vi "RFmx Analysis Only Sanity Check.vi"() -> ()   [LabVIEW 2017]
uses:
  <vilib>/Utility/error.llb/DialogType.ctl
  <vilib>/RFmx/SpecAn/mx/RFmxSpecAn.llb/RFmxSpecAn Select Measurement (Multiple).vi
  <vilib>/RFmx/SpecAn/mx/RFmxSpecAn.llb/RFmxSpecAn Analyze (IQ).vi
  <vilib>/RFmx/SpecAn/mx/RFmxSpecAn.llb/RFmxSpecAn CHP Fetch Measurement.vi
  <vilib>/RFmx/SpecAn/mx/RFmxSpecAn.llb/RFmxSpecAn TXP Fetch Power Trace.vi
  <vilib>/RFmx/SpecAn/mx/RFmxSpecAn.llb/RFmxSpecAn CHP Fetch Spectrum.vi
  <resource>/objmgr/RFmxInstr.rc
panel:
  out "Numeric Control":i32
  out "Waveform Graph":cluster{"x0":dbl, "dx":dbl, "y":sgl[]}(graph)
  in  "Enum":enum16{"Correct Behavior", "Incorrect Behavior"}(ring)
  out "Absolute Power (dBm)":dbl format="%.2f"
  out "Recommended Min Sample Rate (Hz)":dbl format="%#_6p"
  out "Recommended Acquisition Time (s)":dbl format="%#_6p"
  out "Waveform Graph 2":cluster{"x0":dbl, "dx":dbl, "y":sgl[]}(graph)
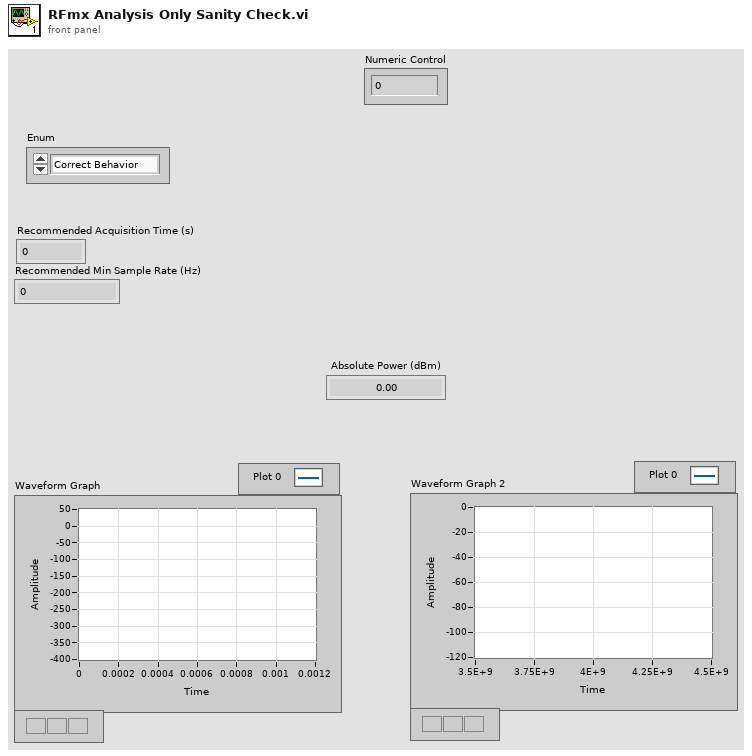
[diagram p1: front panel]
types:
  T1 = typedef "DialogType.ctl" = u16
  T2 = enum16{"open", "open or create", "create or replace", "create", "open (read-only)"}
  T3 = enum16{"ACP", "CCDF", "CHP", "FCnt", "Harmonics", "OBW", "SEM", "Spectrum", "Spur", "TXP", "AMPM", "DPD", "IQ", "IM", "NF", "PhaseNoise"}[]
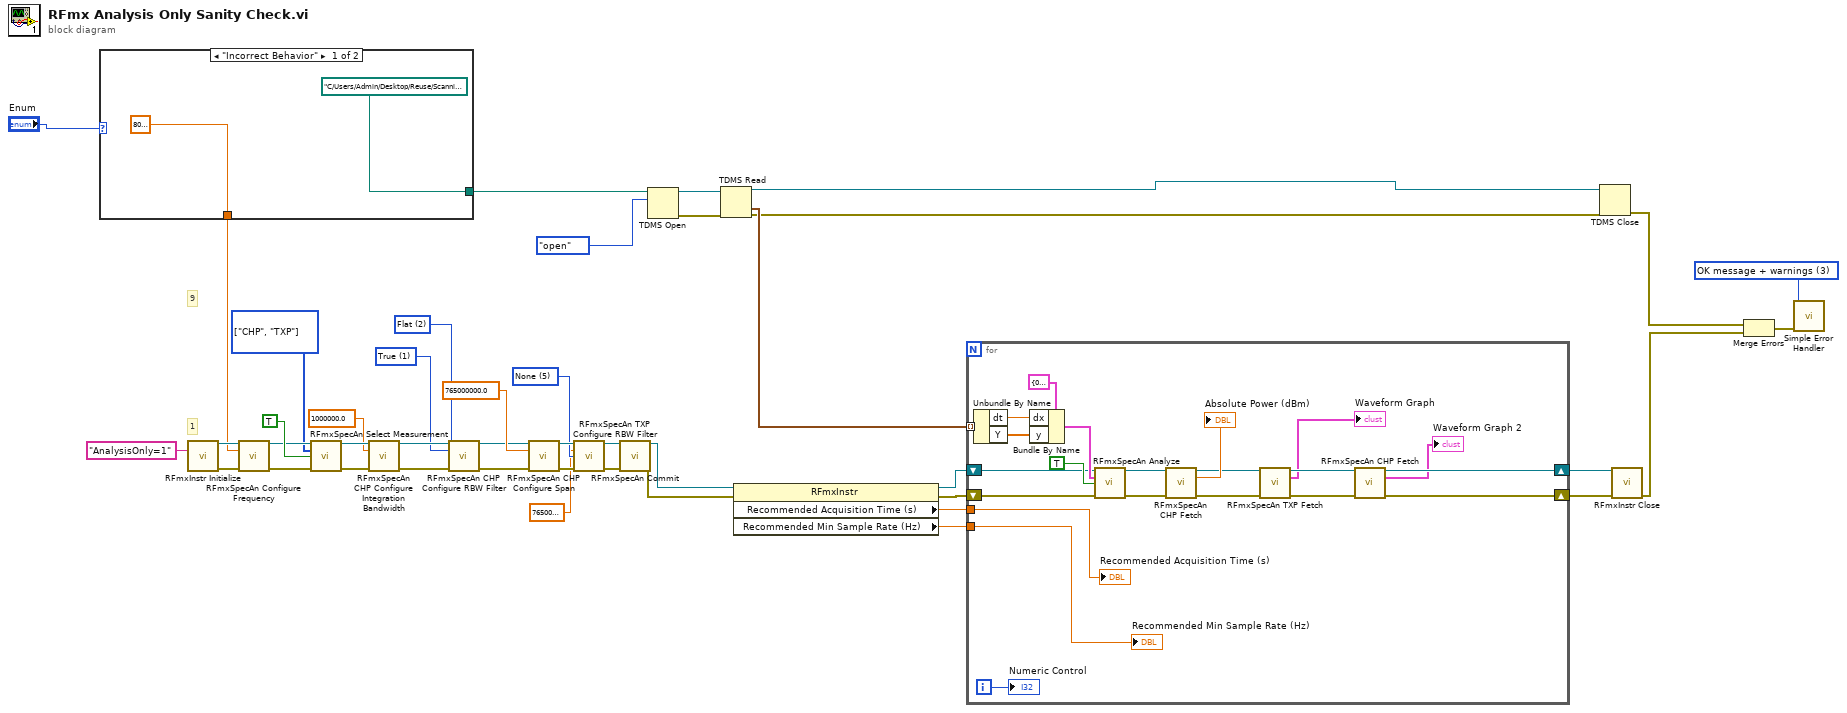
[diagram p0: block diagram]
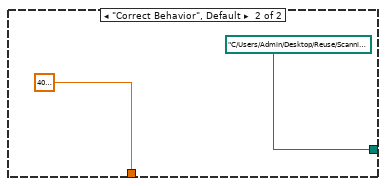
[diagram p2: hidden frame]
diagram:
  w1 = 2 items=["FFT Based", "Gaussian", "Flat"] ("RBW Filter Type")
  w2 = 1 items=["False", "True"] ("RBW Auto")
  w7 = 5 items=["None"=5, "Gaussian"=1, "Flat"=2, "RRC"=6] ("RBW Filter Type")
  w14 = T1 3 items=["no dialog", "OK message", "continue or stop message", "OK message + warnings", "continue/stop + warnings"] ("type of dialog (OK msg:1)")
  w25 = T3 [enum."CHP", enum."TXP"] items=["ACP", "CCDF", "CHP", "FCnt", "Harmonics", "OBW", "SEM", "Spectrum", "Spur", "TXP", "AMPM", "DPD", "IQ", "IM", "NF", "PhaseNoise"] ("Measurements")
  # "9"
  # "1"
  n1 = case shown="\"Incorrect Behavior\"" "Enum" {
    tunnel: [8000000000.0 ("Center Frequency (Hz)") 4000000000.0 ("Center Frequency (Hz)")] -> w26
    tunnel: [path "C:/Users/Admin/Desktop/Reuse/Scanning Speed PXIe 5668/Data8G.tdms.txt.tdms" ("file path") path "C:/Users/Admin/Desktop/Reuse/Scanning Speed PXIe 5668/Data4G.tdms.txt.tdms" ("file path")] -> w11
    frame "Incorrect Behavior" {
    }
    frame "Correct Behavior", Default {
    }
  }
  n2 = call <vilib>:"RFmxInstr Initialize.vi"("Option String"="AnalysisOnly=1") -> ("Instrument Handle Out"=w43:refnum<k21>, "error out"=w42:errorcluster)  [unwired: 12 in, 1 out]
  n3 = call <vilib>:"RFmxSpecAn Configure Frequency.vi"("Instrument Handle In"=w43, "Center Frequency (Hz)"=w26, "error in (no error)"=w42) -> ("Instrument Handle Out"=w40:refnum<k21>, "error out"=w39:errorcluster)  [unwired: 11 in]
  n4 = call-poly <vilib>:"RFmxSpecAn Select Measurement.vi"("Instrument Handle In"=w40, "Measurements"=w25, "Enable All Traces"=TRUE, "error in (no error)"=w39) -> ("Instrument Handle Out"=w38:refnum<k21>, "error out"=w37:errorcluster)  [unwired: 10 in]
  n5 = call <vilib>:"RFmxSpecAn CHP Configure Integration Bandwidth.vi"("Instrument Handle In"=w38, "Integration Bandwidth (Hz)"=1000000.0, "error in (no error)"=w37) -> ("Instrument Handle Out"=w4:refnum<k21>, "error out"=w35:errorcluster)  [unwired: 11 in]
  n6 = call <vilib>:"RFmxSpecAn CHP Configure RBW Filter.vi"("Instrument Handle In"=w4, "RBW Auto"=w2, "RBW Filter Type"=w1, "error in (no error)"=w35) -> ("Instrument Handle Out"=w3:refnum<k21>, "error out"=w5:errorcluster)  [unwired: 10 in]
  n7 = call <vilib>:"RFmxSpecAn CHP Configure Span.vi"("Instrument Handle In"=w3, "Span (Hz)"=765000000.0, "error in (no error)"=w5) -> ("Instrument Handle Out"=w9:refnum<k21>, "error out"=w30:errorcluster)  [unwired: 11 in]
  n8 = call <vilib>:"RFmxSpecAn TXP Configure RBW Filter.vi"("Instrument Handle In"=w9, "RBW (Hz)"=765000000.0, "RBW Filter Type"=w7, "error in (no error)"=w30) -> ("Instrument Handle Out"=w8:refnum<k21>, "error out"=w10:errorcluster)  [unwired: 10 in]
  n9 = call <vilib>:"RFmxSpecAn Commit.vi"("Instrument Handle In"=w8, "error in (no error)"=w10) -> ("Instrument Handle Out"=w27:refnum<k21>, "error out"=w28:errorcluster)  [unwired: 12 in]
  n10 = TDMS Open(10:T2."open" ("operation (0:open)"), 11:w11) -> (0:w21:errorcluster, 3:w20:refnum<k34>)  [unwired: 5 in]
  n11 = TDMS Read(0:w20, 11:w21) -> (4:w12:refnum<k34>, 10:w19:waveform(dbl)[], 15:w18:errorcluster)  [unwired: 6 in, 3 out]
  n12 = property class="RFmxInstr"(reference=w27, error in=w28) -> (reference out=w31:refnum<k21>, error out=w29:errorcluster, "Recommended Acquisition Time (s)"=w24:dbl, "Recommended Min Sample Rate (Hz)"=w23:dbl)
  n13 = for {
    tunnel: w24 -> [w59]
    tunnel: w23 -> [w58]
    tunnel: w19 -> [w57] mode=indexing
    shift-right: [w65] -> w33
    shift-left: w31 -> [w61]
    shift-right: [w63] -> w32
    shift-left: w29 -> [w60]
    i -> [w49]
    n14 = Unbundle By Name(w57) -> ("dt"=w56:dbl, "Y"=w55:dbl[])
    n15 = Bundle By Name(cluster=cluster{"x0":dbl, "dx":dbl, "y":csg[]} {"x0"=0.0, "dx"=0.0, "y"=[]} ("IQ"), "dx"=w56, "y"=w55) -> (w67:cluster{"x0":dbl, "dx":dbl, "y":csg[]})
    n16 = call-poly <vilib>:"RFmxSpecAn Analyze.vi"("Instrument Handle In"=w61, "IQ"=w67, "Reset?"=TRUE, "error in (no error)"=w60) -> ("Instrument Handle Out"=w70:refnum<k21>, "error out"=w69:errorcluster)  [unwired: 8 in, 2 out]
    n17 = call-poly <vilib>:"RFmxSpecAn CHP Fetch.vi"("Instrument Handle In"=w70, "error in (no error)"=w69) -> ("Instrument Handle Out"=w52:refnum<k21>, "Absolute Power (dBm)"=→"Absolute Power (dBm)":dbl, "error out"=w64:errorcluster)  [unwired: 8 in, 3 out]
    n18 = call-poly <vilib>:"RFmxSpecAn TXP Fetch.vi"("Instrument Handle In"=w52, "error in (no error)"=w64) -> ("Instrument Handle Out"=w51:refnum<k21>, "Power (dBm)"=→"Waveform Graph":cluster{"x0":dbl, "dx":dbl, "y":sgl[]}, "error out"=w53:errorcluster)  [unwired: 11 in]
    n19 = call-poly <vilib>:"RFmxSpecAn CHP Fetch.vi"("Instrument Handle In"=w51, "error in (no error)"=w53) -> ("Instrument Handle Out"=w65:refnum<k21>, "Spectrum (dBm)"=→"Waveform Graph 2":cluster{"x0":dbl, "dx":dbl, "y":sgl[]}, "error out"=w63:errorcluster)  [unwired: 11 in]
    "Recommended Acquisition Time (s)" <- w59
    "Recommended Min Sample Rate (Hz)" <- w58
    "Numeric Control" <- w49
  }
  n20 = TDMS Close(8:w18, 11:w12) -> (0:w17:errorcluster)  [unwired: 1 out]
  n21 = call <vilib>:"RFmxInstr Close.vi"("Instrument Handle In"=w33, "error in (no error)"=w32) -> ("error out"=w16:errorcluster)  [unwired: 13 in]
  n22 = Merge Errors(w17, w16) -> (w15:errorcluster)
  n23 = call <vilib>:"Simple Error Handler.vi"("type of dialog (OK msg:1)"=w14, "error in (no error)"=w15) -> ()  [unwired: 3 in, 5 out]
